vi "OpenVS.vi"   [LabVIEW 2013, in "MiscHelperVIs.lvlib"]
uses:
  MiscHelperVIs.lvlib
  <vilib>/Utility/sysdir.llb/System Directory Type.ctl
panel:
  # "This VI calls VeriStand"
types:
  T1 = typedef "System Directory Type.ctl" = i32
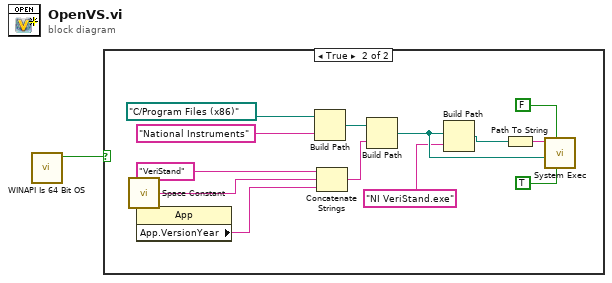
[diagram p0: block diagram]
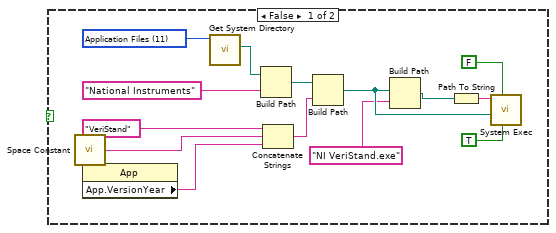
[diagram p2: hidden frame]
diagram:
  n1 = call "WINAPI Is 64 Bit OS.vi"() -> ("Is64Bit"=w1:bool)  [unwired: 10 in, 1 out]
  n2 = case shown="True" w1 {
    frame False {
      w14 = T1 11 items=["User Home"=0, "User Desktop"=1, "User Documents"=2, "User Application Data"=3, "User Preferences"=4, "User Temporary"=5, "Public Documents"=6, "Public Application Data"=7, "Public Preferences"=8, "Public Cache"=13, "System Core Libraries"=9, "System Installed Libraries"=10, "Application Files"=11, "Boot Volume Root"=12] ("system directory type")
      n3 = call <vilib>:"Space Constant.vi"() -> ("String"=w6:string)
      n4 = property class="App"() -> ("App.VersionYear"=w7:string)  [unwired: 2 in, 2 out]
      n5 = call <vilib>:"Get System Directory.vi"("system directory type"=w14) -> ("system directory"=w13:path)  [unwired: 10 in]
      n6 = Build Path(base path=w13, name or relative path="National Instruments") -> (appended path=w11:path)
      n7 = Concatenate Strings("VeriStand" ("name or relative path"), w6, w7) -> (w5:string)
      n8 = Build Path(base path=w11, name or relative path=w5) -> (appended path=w4:path)
      n9 = Build Path(base path=w4, name or relative path="NI VeriStand.exe") -> (appended path=w10:path)
      n10 = Path To String(path=w10) -> (string=w9:string)
      n11 = call <vilib>:"System Exec.vi"("run minimized? (F)"=TRUE, "wait until completion? (T)"=FALSE, "working directory"=w4, "command line"=w9) -> ()  [unwired: 4 in, 4 out]
    }
    frame True {
      n12 = call <vilib>:"Space Constant.vi"() -> ("String"=w21:string)
      n13 = property class="App"() -> ("App.VersionYear"=w22:string)  [unwired: 2 in, 2 out]
      n14 = Build Path(base path=path "C:/Program Files (x86)", name or relative path="National Instruments") -> (appended path=w26:path)
      n15 = Concatenate Strings("VeriStand" ("name or relative path"), w21, w22) -> (w20:string)
      n16 = Build Path(base path=w26, name or relative path=w20) -> (appended path=w19:path)
      n17 = Build Path(base path=w19, name or relative path="NI VeriStand.exe") -> (appended path=w25:path)
      n18 = Path To String(path=w25) -> (string=w24:string)
      n19 = call <vilib>:"System Exec.vi"("run minimized? (F)"=TRUE, "wait until completion? (T)"=FALSE, "working directory"=w19, "command line"=w24) -> ()  [unwired: 4 in, 4 out]
    }
  }
